vi "GetScalerDataV830.vi"(8 "error in (no error)":errorcluster, 10 "handle in":i32, 11 "VME Base Address":u32) -> (0 "error out":errorcluster, 2 "handle out":i32, 3 "Buff":u32[](array[numeric]))   [LabVIEW 2014]
uses:
  Program Files (x86)/CAEN/Comm/labview/CAENComm.lvlib
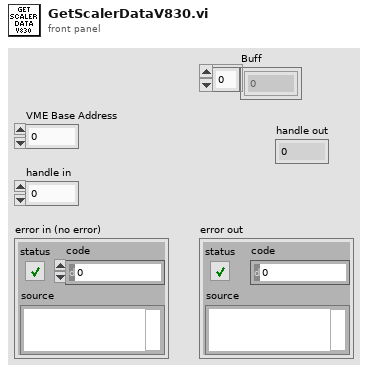
[diagram p1: front panel]
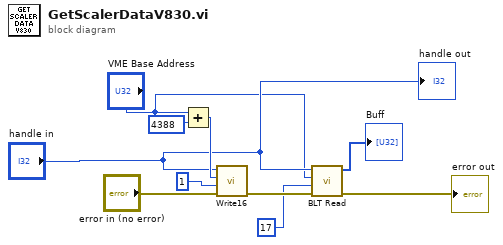
[diagram p0: block diagram]
diagram:
  n1 = Add(x="VME Base Address", y=u32 4388) -> (x+y=w9:u32)
  n2 = call "Write16.vi"("error in (no error)"="error in (no error)", "Data"=u16 1, "Address"=w9, "handle"="handle in") -> ("error out"=w7:errorcluster)  [unwired: 7 in]
  n3 = call "BLT Read.vi"("error in (no error)"=w7, "BltSize"=17, "Address"="VME Base Address", "handle"="handle in") -> ("error out"=→"error out":errorcluster, "Buff"=→"Buff":u32[])  [unwired: 5 in, 1 out]
  "handle out" <- "handle in"
